vi "CANopenPDORead.vi"(0 "FPGA VI Reference In":refnum<k20>, 1 "Node ID":u8, 3 "PDO configuration":T1, 5 "error in":errorcluster) -> (4 "ID":u32, 6 "FPGA VI Reference Out":refnum<k20>, 7 "Boolean array":bool[](array[boolean]), 8 "error out":errorcluster)   [LabVIEW 2016]
doc: "This VI updates the configured PDO memory for a particular COB ID. On first call it starts the periodic transmit process."
uses:
  <vilib>/rvi/errors/niLvFpgaAdjustHostInterfaceError.vi
  <vilib>/Utility/error.llb/Error Cluster From Error Code.vi
  <vilib>/rvi/interface/nirviReadWriteControl/nirviReadWriteControl.xnode
  FPGA Bitfiles/EV-MCU_FPGATarget_CANEngine(FPGA)b_eM8Xz3qYJVA.lvbitx
  CAN_Engine(FPGA)_basic.vi
  NiFpgaLv.dll
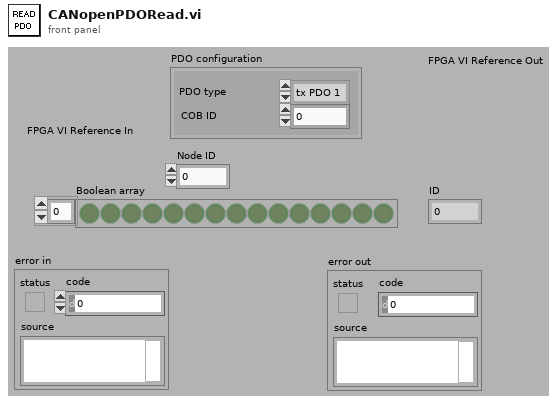
[diagram p1: front panel]
types:
  T1 = cluster{"PDO type":enum8{"tx PDO 1", "tx PDO 2", "tx PDO 3", "tx PDO 4"}, "COB ID":u32}
  T2 = enum8{"tx PDO 1", "tx PDO 2", "tx PDO 3", "tx PDO 4"}
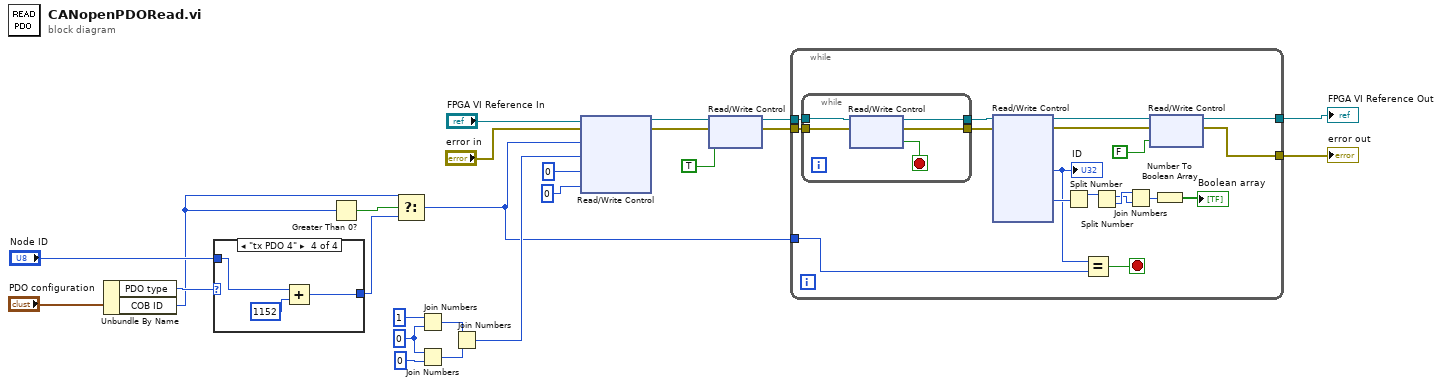
[diagram p0: block diagram]
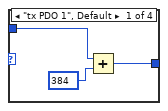
[diagram p2: hidden frame]
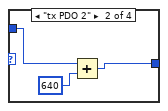
[diagram p3: hidden frame]
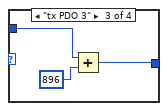
[diagram p4: hidden frame]
diagram:
  w22 = u8 0 ("lo")
  n1 = Unbundle By Name("PDO configuration") -> ("PDO type"=w9:T2, "COB ID"=w6:u32)
  n2 = case shown="\"tx PDO 4\"" w9 {
    tunnel: "Node ID" -> [w27 w29 w32 w35]
    tunnel: [w25 w28 w31 w34] -> w5
    frame "tx PDO 1", Default {
      n3 = Add(x=w27, y=u32 384) -> (x+y=w25:u32)
    }
    frame "tx PDO 2" {
      n4 = Add(x=w29, y=u32 640) -> (x+y=w28:u32)
    }
    frame "tx PDO 3" {
      n5 = Add(x=w32, y=u32 896) -> (x+y=w31:u32)
    }
    frame "tx PDO 4" {
      n6 = Add(x=w35, y=u32 1152) -> (x+y=w34:u32)
    }
  }
  n7 = Greater Than 0?(x=w6) -> (x > 0?=w7:bool)
  n8 = Select(t=w6, s=w7, f=w5) -> (s? t:f=w1:u32)
  n9 = Join Numbers(hi=u8 1, lo=w22) -> ((hi.lo)=w24:u16)
  n10 = Join Numbers(hi=w22, lo=u8 0) -> ((hi.lo)=w23:u16)
  n11 = Join Numbers(hi=w24, lo=w23) -> ((hi.lo)=w2:u32)
  n12 = xnode "Read/Write Control"("FPGA VI Reference In"="FPGA VI Reference In", "error in"="error in", "U32 Out 3"=w1, "U32 Out 4"=w2, "U32 Out 5"=u32 0 ("element"), "U32 Out 6"=u32 0 ("element")) -> ("FPGA VI Reference Out"=w19:refnum<k20>, "error out"=w18:errorcluster)
  n13 = xnode "Read/Write Control"("FPGA VI Reference In"=w19, "error in"=w18, "Write"=TRUE) -> ("FPGA VI Reference Out"=w13:refnum<k20>, "error out"=w12:errorcluster)
  n14 = while {
    tunnel: w13 -> [w54]
    tunnel: w12 -> [w53]
    tunnel: [w41] -> w4
    tunnel: [w40] -> w3
    tunnel: w1 -> [w38]
    stop <- w37 stop-if-true
    n15 = while {
      tunnel: w53 -> [w59]
      tunnel: w54 -> [w58]
      tunnel: [w56] -> w43
      tunnel: [w55] -> w42
      stop <- w57 stop-if-true
      n16 = xnode "Read/Write Control"("FPGA VI Reference In"=w58, "error in"=w59) -> ("FPGA VI Reference Out"=w55:refnum<k20>, "error out"=w56:errorcluster, "Ready"=w57:bool)
    }
    n17 = xnode "Read/Write Control"("FPGA VI Reference In"=w42, "error in"=w43) -> ("FPGA VI Reference Out"=w49:refnum<k20>, "error out"=w50:errorcluster, "U32 In 3"=w39:u32, "U32 In 5"=w52:u32)  [unwired: 4 out]
    "ID" <- w39
    n18 = Split Number(x=w52) -> (hi(x)=w48:u16)  [unwired: 1 out]
    n19 = Equal?(x=w39, y=w38) -> (x = y?=w37:bool)
    n20 = Split Number(x=w48) -> (hi(x)=w46:u8, lo(x)=w47:u8)
    n21 = Join Numbers(hi=w47, lo=w46) -> ((hi.lo)=w45:u16)
    n22 = xnode "Read/Write Control"("FPGA VI Reference In"=w49, "error in"=w50, "Ready"=FALSE ("Read")) -> ("FPGA VI Reference Out"=w41:refnum<k20>, "error out"=w40:errorcluster)
    n23 = Number To Boolean Array(number=w45) -> (Boolean array=→"Boolean array":bool[])
  }
  "error out" <- w3
  "FPGA VI Reference Out" <- w4
